vi "get event.vi"(8 "error in":errorcluster, 11 "module in":refnum<class "TBM module execution interface.lvclass">) -> (0 "error out":errorcluster, 1 "elements remaining":i32, 2 "event":T1, 3 "module out":refnum<class "TBM module execution interface.lvclass">)   [LabVIEW 2013, in "TBM module execution interface.lvclass"]
uses:
  TBM module execution interface.lvclass
  <vilib>/NI/Tag Bus/events/event.ctl
  TBM module execution interface.lvclass/TBM module execution interface.ctl
  <vilib>/NI/Tag Bus/events/data bus events.lvlib
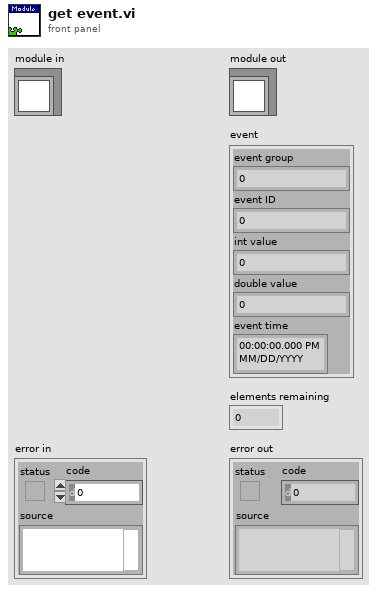
[diagram p1: front panel]
types:
  T1 = typedef "data bus events.lvlib/event.ctl" = cluster{"event group":i64, "event ID":i64, "int value":i64, "double value":dbl, "event time":timestamp}
  T2 = typedef "data bus events.lvlib/event queue.ctl" = cluster{"head":i32, "count":i32, "event array":T1[]}
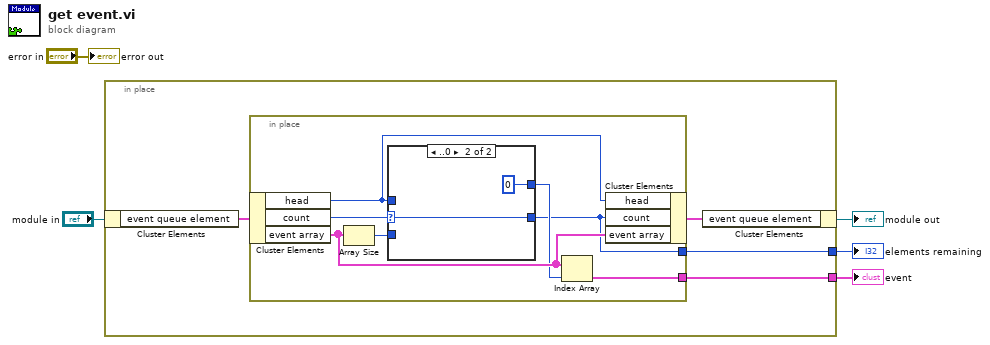
[diagram p0: block diagram]
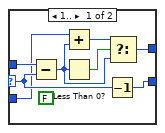
[diagram p2: hidden frame]
diagram:
  n1 = in-place {
    in-place-border: [w9] -> w5
    in-place-border: [w6] -> w1
    n2 = in-place-cluster #1("module in") -> ("event queue element"=w8:T2)
    n3 = in-place {
      in-place-border: [w15] -> w9
      in-place-border: [w10] -> w6
      n4 = in-place-cluster #2(w8) -> ("head"=w12:i32, "count"=w16:i32, "event array"=w14:T1[])
      n5 = Array Size(array=w14) -> (size(s)=w13:i32)
      n6 = case shown="..0" w16 {
        selector: w16 -> [w22 w26]
        tunnel: w12 -> [w23 _]
        tunnel: [w24 w26] -> w10
        tunnel: w13 -> [w20 _]
        tunnel: [w17 0] -> w11
        frame 1.. {
          (unwired) FALSE
          n7 = Subtract(x=w23, y=w22) -> (x-y=w18:i32)
          n8 = Add(x=w20, y=w18) -> (x+y=w19:i32)
          n9 = Less Than 0?(x=w18) -> (x < 0?=w21:bool)
          n10 = Decrement(x=w22) -> (x-1=w24:i32)
          n11 = Select(t=w19, s=w21, f=w18) -> (s? t:f=w17:i32)
        }
        frame ..0 {
        }
      }
      n12 = Index Array(array=w14, index=w11) -> (element=w15:T1)
      n13 = in-place-cluster #2("head"=w12, "count"=w10, "event array"=w14) -> (w7:T2)
    }
    n14 = in-place-cluster #1("event queue element"=w7) -> (→"module out":refnum<class "TBM module execution interface.lvclass">)
  }
  "event" <- w5
  "elements remaining" <- w1
  "error out" <- "error in"
